vi "tcpServerCallBack.vi"(8 "error in (no error)":errorcluster, 11 "TcpServerCmd in":refnum<class "TcpServerCmd.lvclass">) -> (0 "error out":errorcluster, 3 "TcpServerCmd out":refnum<class "TcpServerCmd.lvclass">)   [LabVIEW 2018, in "TcpServerCmd.lvclass"]
doc: "Receive the incoming json command from TCP Client and process it, and send the results as an user event to the LabVIEW Component.\n\nPut the VI in preallocated reentrant clone execution."
uses:
  TcpServerCmd.lvclass
  home/pcortes/Documents/github/ts_labview_tcp_json/src/TcpServerBase/TcpServerBase.lvclass
  TcpServerBase/TcpServerBase.lvclass/TcpServerBase.ctl
  TcpServerCmd.lvclass/TcpServerCmd.ctl
  TcpServerBase/TcpServerBase.lvclass
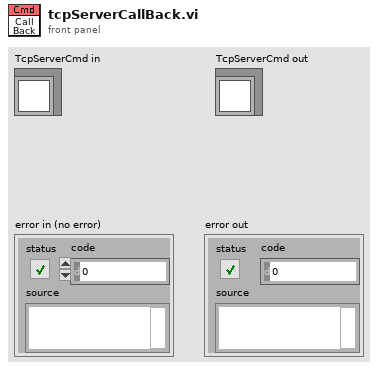
[diagram p1: front panel]
types:
  T1 = cluster{"connection ID":refnum<k5>, "firstConnection":bool}
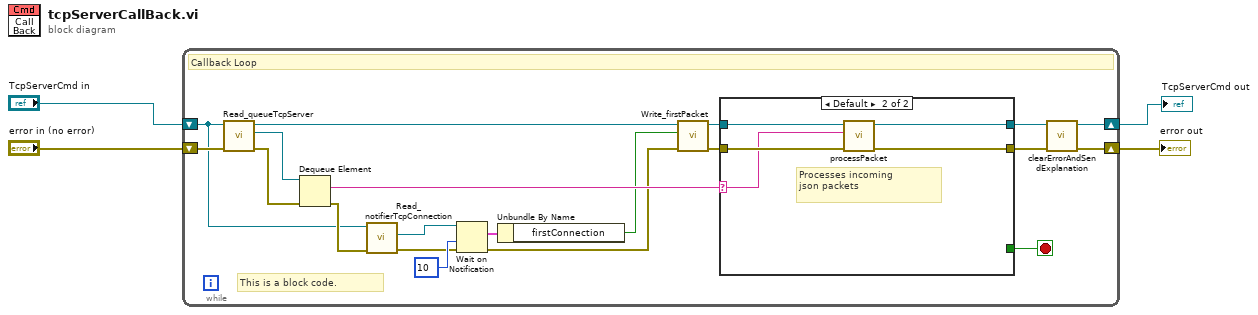
[diagram p0: block diagram]
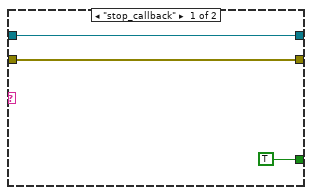
[diagram p2: hidden frame]
diagram:
  n1 = while {
    shift-right: [w11] -> w4
    shift-left: "error in (no error)" -> [w23]
    shift-right: [w9] -> w1
    shift-left: "TcpServerCmd in" -> [w5]
    stop <- w12 stop-if-true
    # "This is a block code."
    # "Callback Loop"
    n2 = call "Read_queueTcpServer.vi"("error in (no error)"=w23, "TcpServerBase in"=w5) -> ("error out"=w19:errorcluster, "queueTcpServer"=w24:refnum<queue>, "TcpServerBase out"=w21:refnum<class "TcpServerCmd.lvclass">)  [unwired: 7 in]
    n3 = Dequeue Element(queue=w24, error in (no error)=w19) -> (element=w20:string, error out=w8:errorcluster)  [unwired: 1 in, 2 out]
    n4 = call "Read_notifierTcpConnection.vi"("error in (no error)"=w8, "TcpServerBase in"=w5) -> ("error out"=w7:errorcluster, "notifierTcpConnection"=w6:refnum<notifier>)  [unwired: 7 in, 1 out]
    n5 = Wait on Notification(notifier=w6, timeout in ms (-1)=10, error in (no error)=w7) -> (notification=w15:T1, error out=w13:errorcluster)  [unwired: 1 in, 2 out]
    n6 = Unbundle By Name(w15) -> ("firstConnection"=w14:bool)
    n7 = call "Write_firstPacket.vi"("error in (no error)"=w13, "firstPacket"=w14, "TcpServerCmd in"=w21) -> ("error out"=w17:errorcluster, "TcpServerCmd out"=w18:refnum<class "TcpServerCmd.lvclass">)  [unwired: 7 in]
    n8 = case shown="Default" w20 {
      selector: w20 -> [_ w28]
      tunnel: w18 -> [w26 w32]
      tunnel: [TRUE _] -> w12
      tunnel: [w25 w31] -> w22
      tunnel: [w26 w30] -> w10
      tunnel: w17 -> [w25 w29]
      frame "stop_callback" {
      }
      frame Default {
        # "Processes incoming\njson packets"
        n9 = call "processPacket.vi"("error in (no error)"=w29, "tcpPacket"=w28, "tcpServerCmd in"=w32) -> ("error out"=w31:errorcluster, "tcpServerCmd out"=w30:refnum<class "TcpServerCmd.lvclass">)  [unwired: 7 in]
      }
    }
    n10 = call "clearErrorAndSendExplanation.vi"("error in (no error)"=w22, "TcpServerBase in"=w10) -> ("error out"=w11:errorcluster, "TcpServerBase out"=w9:refnum<class "TcpServerCmd.lvclass">)  [unwired: 8 in]
  }
  "error out" <- w4
  "TcpServerCmd out" <- w1
